vi "Insight_RW_ClockRate.vi"(7 "Parameter Type":enum16{"Value", "MAXimum", "MINimum", "DEFault"}(ring), 8 "error in (no error)":errorcluster, 9 "Mode (Read / Write)":enum8{"Write", "Read"}(ring), 10 "Clock Rate (MHz)":dbl=400.0, 11 "telnet connection":T1) -> (0 "error out":errorcluster, 1 "response data":string, 2 "Clock Rate (MHz)":dbl, 3 "telnet  connection out":T1)   [LabVIEW 2015]
doc: "Insight Photonic Solutions\n\nThis VI reads or writes the clock rate for the user sample clock. \n\nNOTE: changing the User Sample Clock Rate from the Laser Drive Clock rate (typically 400 MHz) requires careful decimation of the user's raw data set to properly use the Data Valid Vector (DVV) for the locations of laser hold points. Contact Insight Photonic Solutions for further details.\n\n\nINPUTS\n\nMode - Tells the VI whether the command is a Read or a Write. (Default = Read).\nParameter Type - Tells the VI whether the command should use a Value or a keyword MAXimum, MINimum or DEFault to set the parameter value. (Default = Value).\nClock Rate (MHz) - The numeric value to set the user sample clock rate. (Default = 400.0).\nerror in - The standard LabView Error cluster. Use this to enforce sequentiality and error tracking.\n\nOUTPUTS\n\nresponse data - the complete response string from the laser\nClock Rate (MHz) - the User Sample Clock Rate written to or read from the laser\nerror out - the standard error cluster. Reports errors in reading or writing to the laser, or passes through errors from before this VI.\n\n\nver 1.0 - original release\nver 1.1 - added response data buffer as an output\nver 3.6.2 - added Max/Min/Default support, fixed syntax error, added response parsing"
uses:
  Telnet Session.ctl
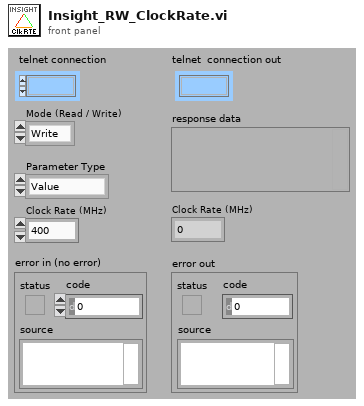
[diagram p1: front panel]
types:
  T1 = typedef "Telnet Session.ctl" = refnum<k1>
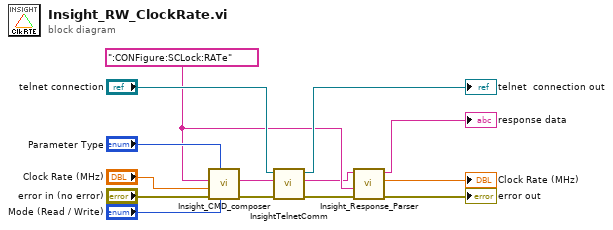
[diagram p0: block diagram]
diagram:
  w2 = ":CONFigure:SCLock:RATe" ("String")
  n1 = call "Insight_CMD_composer.vi"("Mode (Read / Write)"="Mode (Read / Write)", "Parameter Type"="Parameter Type", "error in (no error)"="error in (no error)", "Value"="Clock Rate (MHz)", "CMD"=w2) -> ("error out"=w11:errorcluster, "Command String"=w7:string)  [unwired: 5 in]
  n2 = call "InsightTelnetComm.vi"("error in"=w11, "write buffer (\"\")"=w7, "telnet connection"="telnet connection") -> ("error out"=w4:errorcluster, "response data"=w1:string, "telnet  connection out"=→"telnet  connection out":T1)  [unwired: 4 in]
  n3 = call "Insight_Response_Parser.vi"("error in (no error)"=w4, "Command String"=w2, "Laser Response In"=w1) -> ("error out"=→"error out":errorcluster, "Value"=→"Clock Rate (MHz)":dbl, "Laser Response Out"=→"response data":string)  [unwired: 6 in]
